vi "replace reservation node.vi"(7 "channel type":T2, 8 "error in (no error)":errorcluster, 9 "index of element":i32, 10 "Client Node Ref":T1 format="%.0x", 11 "Item Ref in":T1 format="%.0x") -> (0 "error out":errorcluster, 3 "Item Ref out":T1 format="%.0x")   [LabVIEW 2016]
uses:
  <vilib>/NI Veristand/Custom Device API/Custom Device Item Ref.ctl
  FPGA-Addon/Source/System Explorer/SubVIs/Channel Type.ctl
  <vilib>/NI Veristand/Custom Device API/Get Item Property (Variant).vi
  <vilib>/NI Veristand/Custom Device API/Set Item Property (Variant).vi
  <vilib>/NI VeriStand/Custom Device API/Custom Device API.lvlib
  FPGA-Addon/Source/System Explorer/FPGA Addon System Explorer.lvlib
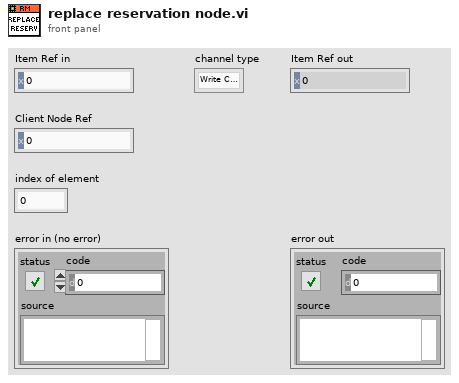
[diagram p1: front panel]
types:
  T1 = typedef "Custom Device API.lvlib/Custom Device Item Ref.ctl" = u64
  T2 = typedef "FPGA Addon System Explorer.lvlib/Channel Type.ctl" = enum16{"Write Channel", "Read Channel", "Write Waveform", "Read Waveform"}
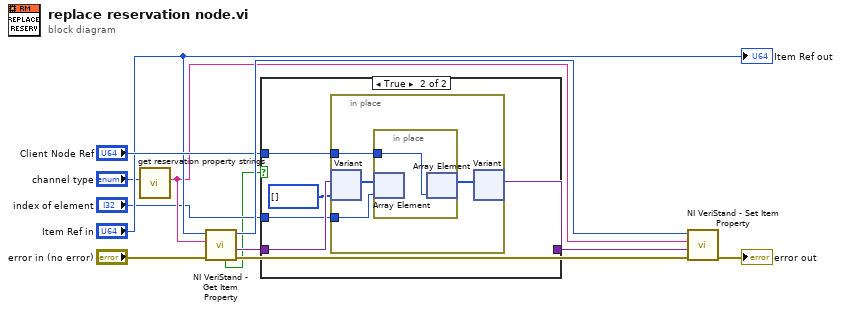
[diagram p0: block diagram]
diagram:
  n1 = call "get reservation property strings.vi"("channel type"="channel type") -> ("reservations"=w5:string)  [unwired: 8 in, 2 out]
  n2 = call-poly <vilib>:"NI VeriStand - Get Item Property.vi"("error in (no error)"="error in (no error)", "Property Name"=w5, "Item Ref in"="Item Ref in") -> ("error out"=w8:errorcluster, "Value"=w4:variant, "Item Ref out"=w12:T1, "Found?"=w1:bool)  [unwired: 5 in]
  n3 = case shown="True" w1 {
    tunnel: "Client Node Ref" -> [_ w18]
    tunnel: w4 -> [w13 w17]
    tunnel: "index of element" -> [_ w15]
    tunnel: [w13 w14] -> w2
    frame False {
    }
    frame True {
      n4 = in-place {
        in-place-border: w18 -> [w20]
        in-place-border: w15 -> [w21]
        n5 = in-place-variant #1(w17, T1[] [] ("Client Node Ref")) -> (w22:T1[])  [unwired: 1 out]
        n6 = in-place {
          in-place-border: w20 -> [w23]
          n7 = in-place-array #2(w22, w21) -> ()  [unwired: 1 out]
          n8 = in-place-array #2(w23) -> (w19:T1[])  [unwired: 1 out]
        }
        n9 = in-place-variant #1(w19) -> (w14:variant)  [unwired: 1 out]
      }
    }
  }
  n10 = call-poly <vilib>:"NI VeriStand - Set Item Property.vi"("error in (no error)"=w8, "Value"=w2, "Property Name"=w5, "Item Ref in"=w12) -> ("error out"=→"error out":errorcluster)  [unwired: 5 in, 2 out]
  "Item Ref out" <- "Item Ref in"
